vi "Connect.vi"(8 "error in (no error)":errorcluster, 11 "MQTT In":refnum<class "MQTT Client.lvclass">) -> (0 "error out":errorcluster, 3 "MQTT Out":refnum<class "MQTT Client.lvclass">)   [LabVIEW 2020, in "MQTT Client.lvclass"]
uses:
  MQTT Client.lvclass
  mqttCmd/mqttCmdConnect/ConnectMqttMsg.lvclass
  C:/Projects/Libraries/Gore SM 2020/mqtt-LabVIEW/src/class/mqtt/mqttCmd/BaseMqttMsg.lvclass
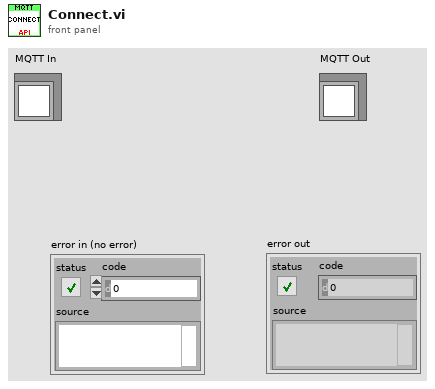
[diagram p1: front panel]
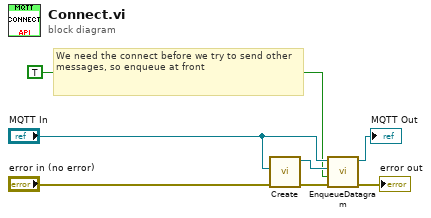
[diagram p0: block diagram]
diagram:
  # "We need the connect before we try to send other messages, so enqueue at front"
  n1 = call "Create.vi"("error in (no error)"="error in (no error)", "mqtt instance"="MQTT In") -> ("error out"=w4:errorcluster, "mqttCmdConnect out"=w3:refnum<class "ConnectMqttMsg.lvclass">)  [unwired: 8 in]
  n2 = call "EnqueueDatagram.vi"("error in (no error)"=w4, "Enqueue at Front? (F)"=TRUE, "mqttCmd"=w3, "mqtt in"="MQTT In") -> ("error out"=→"error out":errorcluster, "mqtt out"=→"MQTT Out":refnum<class "MQTT Client.lvclass">)  [unwired: 6 in]
